vi "Waveform - Scalar Limit Comparison.vi"() -> ()   [LabVIEW 2020]
doc: "Shows how to determine if the waveform has values that do not satisfy a user defined condition."
panel:
  in  "Limit":dbl=50.0
  out "Graph":waveform(dbl)[](graph)
  # "Overview: Compares the data values of a waveform against a limit value with the Waveform Scalar Limit Comparison VI.\nInstructions:\n1. Specify a Limit value.\n2. Run the VI. All values in the waveform that are less than the specified Limit will appear in the passed plot."
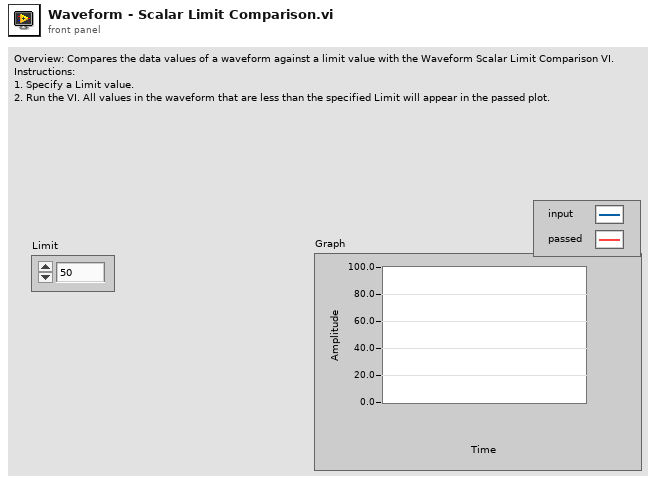
[diagram p1: front panel]
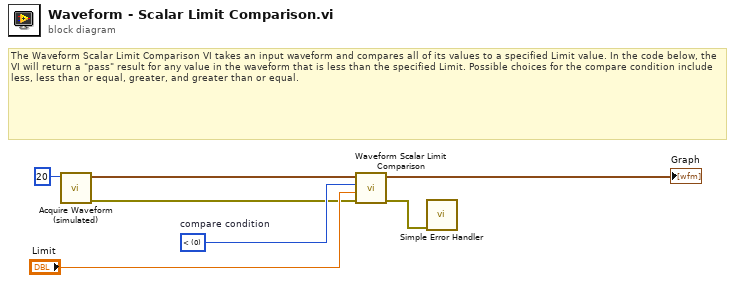
[diagram p0: block diagram]
diagram:
  w3 = u16 0 items=["<", "<=", ">", ">="]  # compare condition
  # "The Waveform Scalar Limit Comparison VI takes an input waveform and compares all of its values to a specified Limit value. In the code below, the VI will return a \"pass\" result for any value in the waveform that is less than the specified Limit. Possible choices for the compare condition include less, less than or equal, greater, and greater than or equal."
  n1 = call "Acquire Waveform (simulated).vi"("# points"=20) -> ("error out"=w2:errorcluster, "waveform output"=w5:waveform(dbl))  [unwired: 9 in]
  n2 = call <vilib>:"Waveform Scalar Limit Comparison.vi"("error in (no error)"=w2, "limit"="Limit", "compare condition"=w3, "data"=w5) -> ("error out"=w1:errorcluster, "output waveforms"=→"Graph":waveform(dbl)[])  [unwired: 5 in, 1 out]
  n3 = call <vilib>:"Simple Error Handler.vi"("error in (no error)"=w1) -> ()  [unwired: 4 in, 5 out]
